vi "Page_Destination_Initialize.vi"(8 "error in (no error)":errorcluster, 9 "ctlReferences":T1, 11 "AB_DepDLL in":refnum<class "AB_DepDLL.lvclass">) -> (0 "error out":errorcluster, 3 "AB_DepDLL out":refnum<class "AB_DepDLL.lvclass">)   [LabVIEW 2020, in "AB_DepDLL.lvclass"]
uses:
  <vilib>/AppBuilder/AB_Classes/DepDLL/AB_DepDLL.lvclass
  e:/builds/penguin/labview/branches/2020/dev/dist/vi.lib/AppBuilder/AB_Classes/Build/AB_Build.lvclass
  <resource>/Framework/Providers/Builds/AppBuilder/AB_UI_Page_Destination_References.ctl
  <vilib>/AppBuilder/AB_Classes/DLL/AB_DLL.lvclass
  <vilib>/AppBuilder/AB_Classes/Deployment/AB_Deployment.lvlib
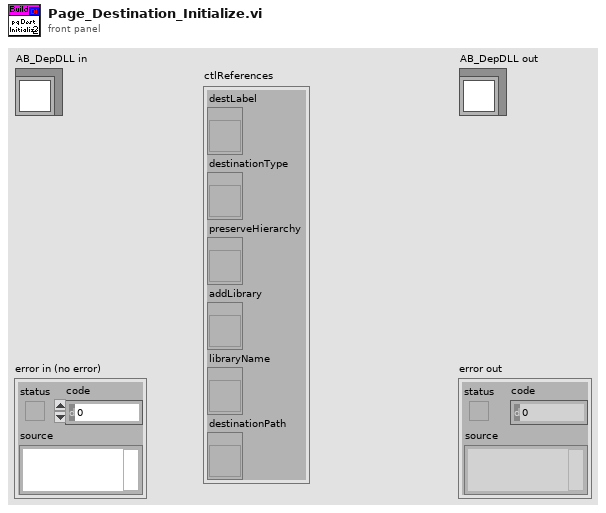
[diagram p1: front panel]
types:
  T1 = typedef "AB_UI_Page_Destination_References.ctl" = cluster{"destLabel":refnum<vi>, "destinationType":refnum<vi>, "preserveHierarchy":refnum<vi>, "addLibrary":refnum<vi>, "libraryName":refnum<vi>, "destinationPath":refnum<vi>}
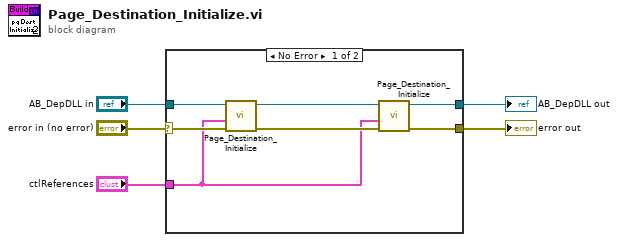
[diagram p0: block diagram]
diagram:
  n1 = case shown="No Error" "error in (no error)" {
    selector: "error in (no error)" -> [w11 w14]
    tunnel: [w7 w14] -> w4
    tunnel: [w9 w13] -> w3
    tunnel: "ctlReferences" -> [w6 _]
    tunnel: "AB_DepDLL in" -> [w12 w13]
    frame No Error {
      n2 = call-parent <vilib>:"Page_Destination_Initialize.vi"("error in (no error)"=w11, "ctlReferences"=w6, "AB_Build in"=w12) -> ("error out"=w8:errorcluster, "AB_Build out"=w10:refnum<class "AB_DepDLL.lvclass">)  [unwired: 7 in]
      n3 = call <vilib>:"Page_Destination_Initialize.vi"("error in (no error)"=w8, "ctlReferences"=w6, "Build in"=w10) -> ("error out"=w7:errorcluster, "Build out"=w9:refnum<class "AB_DepDLL.lvclass">)  [unwired: 7 in]
    }
    frame Error {
    }
  }
  "error out" <- w4
  "AB_DepDLL out" <- w3
